vi "AutomatedStart.vi"() -> ()   [LabVIEW 2014]
uses:
  <vilib>/userdefined/High Color/nirio_resource_hc.ctl
  TriggerChannel.ctl
  <vilib>/FPGAPlugInAG/PCI-7813R/niLvFpga_Open_PCI-7813R.vi
  <vilib>/rvi/interface/nirviOpenFPGA/nirviOpenFPGA.xnode
  FPGA Bitfiles/W7XBolo2017_FPGATarget_fmain2014_9xlV3GyHFfo.lvbitx
  f_main_2014.vi
panel:
  out "error out":errorcluster
  out "Operation Watchdog":bool
  out "No. of Software Triggers \ndetected":dbl
  out "No. of Hardware Triggers \ndetected":dbl
  out "Autmated Start Loop Counter \n(Increasing every 1s)":i32
  out "Timeout ? \n(1s-10s?)":bool
  out "Hardware Trigger \ndetected":bool
  in  "Software Trigger\n(Switch until released)":bool
  in  "Stopp Button":bool
  # "Automated Start W7-X Bolometer DAQ"
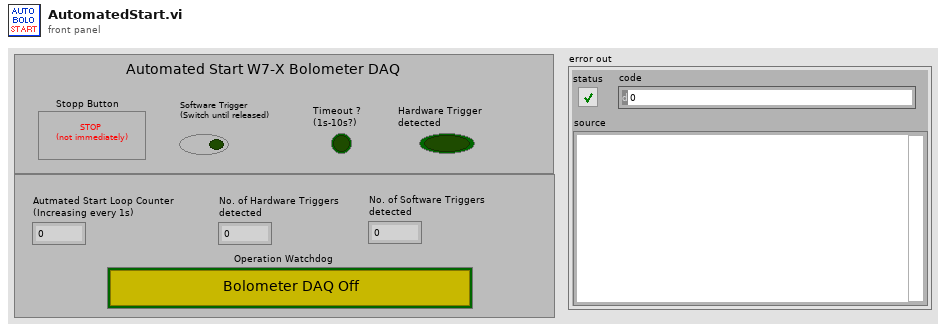
[diagram p1: front panel]
types:
  T1 = typedef "TriggerChannel.ctl" = enum16{"board0 (broken)", "board1 (t = -60sec)", "board2 (t = 0sec)"}
  T2 = enum32{"Invalid", "Standard", "Closed", "Hidden", "Minimized", "Maximized"}
  T3 = typedef "nirio_resource_hc.ctl" = tag
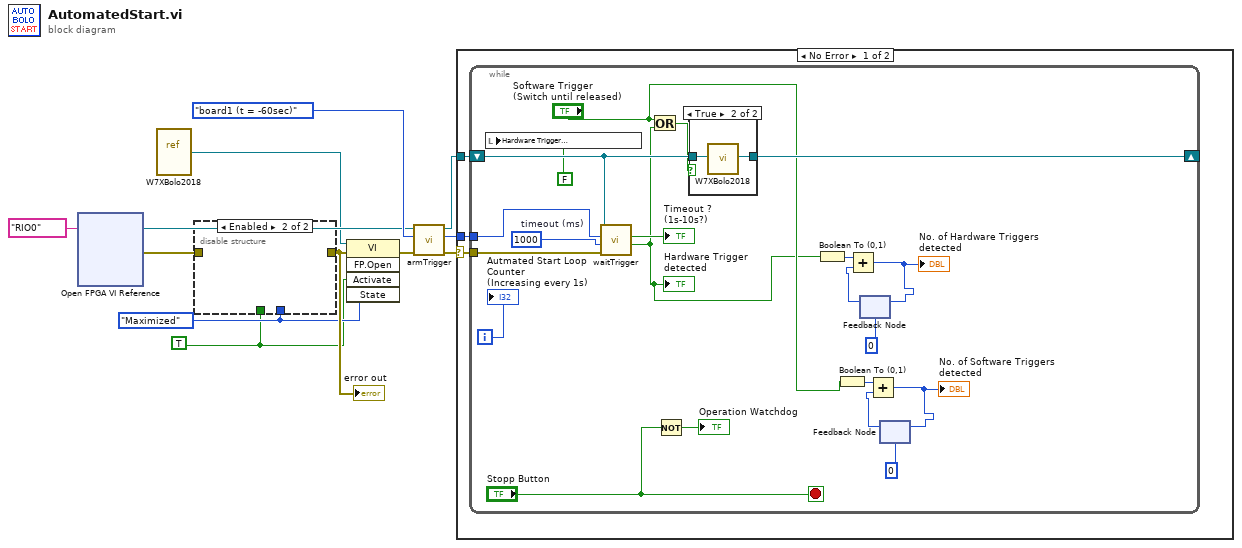
[diagram p0: block diagram]
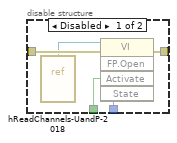
[diagram p2: hidden frame]
diagram:
  w2 = T2."Maximized" ("State")
  w1 = TRUE ("Activate?")
  n1 = xnode "Open FPGA VI Reference"("resource name"=T3 "RIO0") -> ("FPGA VI Reference Out"=w8:refnum<k20>, "error out"=w4:errorcluster)  [unwired: 1 in]
  n2 = vi-ref "W7XBolo2018.vi"() -> (w5:refnum<vi>)
  n3 = disable-structure shown="Enabled" {
    disable-tunnel: w4 -> [w17 _]
    disable-tunnel: [w16 _] -> w3
    disable-tunnel: w2 -> [w15 _]
    disable-tunnel: w1 -> [w14 _]
    frame Disabled {
      n4 = vi-ref "hReadChannels-UandP-2018.vi"() -> (w13:refnum<vi>)
      n5 = invoke class="VI" method="FP.Open"(reference=w13, error in=w17, "Activate"=w14, "State"=w15) -> (error out=w16:errorcluster)  [unwired: 1 in, 4 out]
    }
    frame Enabled {
    }
  }
  "error out" <- w3
  n6 = invoke class="VI" method="FP.Open"(reference=w5, error in=w3, "Activate"=w1, "State"=w2) -> (error out=w11:errorcluster)  [unwired: 1 in, 4 out]
  n7 = call "armTrigger.vi"("error in (no error)"=w11, "Trigger default: board0 (t = 0)"=TriggerChannel."board1 (t = -60sec)", "Refnum in"=w8) -> ("error out"=w10:errorcluster, "IRQ"=w6:i32, "Refnum out"=w7:refnum<k20>)  [unwired: 6 in]
  n8 = case shown="No Error" w10 {
    selector: w10 -> [w18 _]
    tunnel: w7 -> [w20 _]
    tunnel: w6 -> [w19 _]
    frame No Error {
      n9 = while {
        shift-right: [w40] -> _
        shift-left: w20 -> [w41]
        tunnel: w19 -> [w38]
        tunnel: w18 -> [w37]
        i -> [w34]
        stop <- "Stopp Button" stop-if-true
        w39 = 1000  # timeout (ms)
        n10 = local write "Hardware Trigger \ndetected"(FALSE) -> ()
        n11 = call "waitTrigger.vi"("error in (no error)"=w37, "timeout (ms) default: 10s"=w39, "IRQ"=w38, "Refnum in"=w41) -> ("Boolean"=w23:bool, "Timed Out"=→"Timeout ? \n(1s-10s?)":bool)  [unwired: 4 in, 2 out]
        "Hardware Trigger \ndetected" <- w23
        n12 = Or(x="Software Trigger\n(Switch until released)", y=w23) -> (x .or. y?=w29:bool)
        n13 = Not(x="Stopp Button") -> (.not. x?=→"Operation Watchdog":bool)
        n14 = case shown="True" w29 {
          tunnel: w41 -> [w42 w44]
          tunnel: [w42 w43] -> w40
          frame False {
          }
          frame True {
            n15 = call "W7XBolo2018.vi"("FPGA VI Reference In"=w44) -> ("FPGA VI Reference Out"=w43:refnum<k20>)
          }
        }
        n16 = Boolean To (0,1)(Boolean=w23) -> (0, 1=w32:i16)
        n17 = Boolean To (0,1)(Boolean="Software Trigger\n(Switch until released)") -> (0, 1=w27:i16)
        n18 = feedback #1(i16 0) -> (w33:i16)
        n19 = Add(x=w32, y=w33) -> (x+y=w30:i16)
        "No. of Hardware Triggers \ndetected" <- w30
        n20 = feedback-in #1(w30) -> ()
        n21 = feedback #2(i16 0) -> (w28:i16)
        n22 = Add(x=w27, y=w28) -> (x+y=w25:i16)
        "No. of Software Triggers \ndetected" <- w25
        n23 = feedback-in #2(w25) -> ()
        "Autmated Start Loop Counter \n(Increasing every 1s)" <- w34
      }
    }
    frame Error {
    }
  }
